vi "Get Library Name.vi"(11 "VI In":string) -> (0 "Found?":bool, 3 "Lib name":string)   [LabVIEW 2019, in "DependencyInspector.lvlib"]
uses:
  DependencyInspector.lvlib
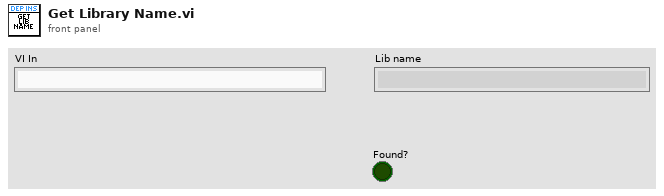
[diagram p1: front panel]
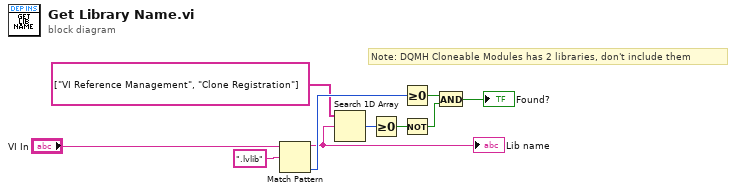
[diagram p0: block diagram]
diagram:
  # "Note: DQMH Cloneable Modules has 2 libraries, don't include them"
  n1 = Match Pattern(string="VI In", regular expression=".lvlib") -> (before substring=w6:string, offset past match=w8:i32)  [unwired: 1 in, 2 out]
  "Lib name" <- w6
  n2 = Search 1D Array(1D array=string[] ["VI Reference Management", "Clone Registration"], element=w6) -> (index of element=w5:i32)  [unwired: 1 in]
  n3 = Greater Or Equal To 0?(x=w5) -> (x >= 0?=w4:bool)
  n4 = Greater Or Equal To 0?(x=w8) -> (x >= 0?=w3:bool)
  n5 = Not(x=w4) -> (.not. x?=w2:bool)
  n6 = And(x=w3, y=w2) -> (x .and. y?=→"Found?":bool)
